vi "Read User Devices.vi"(8 "error in (no error)":errorcluster) -> (0 "error out":errorcluster, 3 "User Devices":refnum<class "Device.lvclass">[](array[class]))   [LabVIEW 2020, in "PicoG-App.lvlib" / "App.lvclass"]
uses:
  App.lvclass
  PicoG-App.lvlib
  <vilib>/Utility/config.llb/NI_LVConfig.lvlib
  <vilib>/Utility/config.llb/Read Key (I32).vi
  Device/Device.lvclass
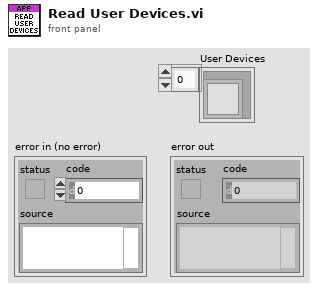
[diagram p1: front panel]
types:
  T1 = typedef "PicoG-App.lvlib/Paths.ctl" = cluster{"User picoG":path, "System picoG":path, "User Config":path, "System Config":path}
  T2 = typedef "NI_LVConfig.lvlib/Config Data RefNum.ctl" = refnum<k1>
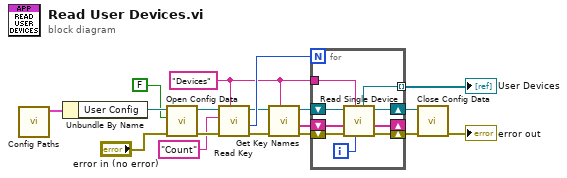
[diagram p0: block diagram]
diagram:
  w1 = "Devices" ("key")
  n1 = call "Config Paths.vi"() -> ("Paths"=w18:T1)  [unwired: 8 in, 3 out]
  n2 = Unbundle By Name(w18) -> ("User Config"=w17:path)
  n3 = call <vilib>:"Open Config Data.vi"("error in (no error)"="error in (no error)", "create file if necessary (T)"=FALSE, "configuration file path"=w17) -> ("error out"=w14:errorcluster, "refnum"=w15:T2)  [unwired: 6 in, 1 out]
  n4 = call-poly <vilib>:"Read Key.vi"("section"=w1, "error in (no error)"=w14, "key"="Count", "refnum"=w15) -> ("error out"=w5:errorcluster, "value"=w12:i32, "refnum out"=w6:T2)  [unwired: 4 in, 1 out]
  n5 = call <vilib>:"Get Key Names.vi"("section"=w1, "error in (no error)"=w5, "refnum"=w6) -> ("error out"=w3:errorcluster, "key names"=w4:string[], "refnum out"=w2:T2)  [unwired: 5 in, 1 out]
  n6 = for {
    N: w12 -> [_]
    shift-right: [w24] -> w9
    shift-left: w3 -> [w26]
    shift-right: [w23] -> w10
    shift-left: w2 -> [w27]
    tunnel: w1 -> [w22]
    tunnel: [w20] -> w11 mode=indexing
    shift-right: [w19] -> _
    shift-left: w4 -> [w21]
    i -> [w25]
    n7 = call "Read Single Device.vi"("Index"=w25, "Section"=w22, "error in (no error)"=w26, "Key Names"=w21, "refnum"=w27) -> ("error out"=w24:errorcluster, "Remaining Key Names"=w19:string[], "refnum out"=w23:T2, "Device"=w20:refnum<class "Device.lvclass">)  [unwired: 3 in]
  }
  "User Devices" <- w11
  n8 = call <vilib>:"Close Config Data.vi"("error in (no error)"=w9, "refnum"=w10) -> ("error out"=→"error out":errorcluster)  [unwired: 8 in, 1 out]
